vi "show_plot_y_axis.vi"(8 "autoscale":bool=TRUE, 11 "plot_ref_in":refnum<vi>) -> (0 "done":bool, 3 "plot_ref_out":refnum<vi>)   [LabVIEW 2025]
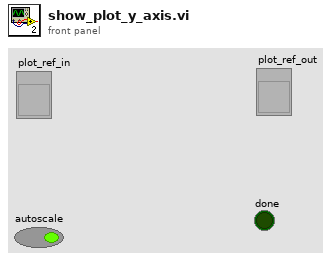
[diagram p1: front panel]
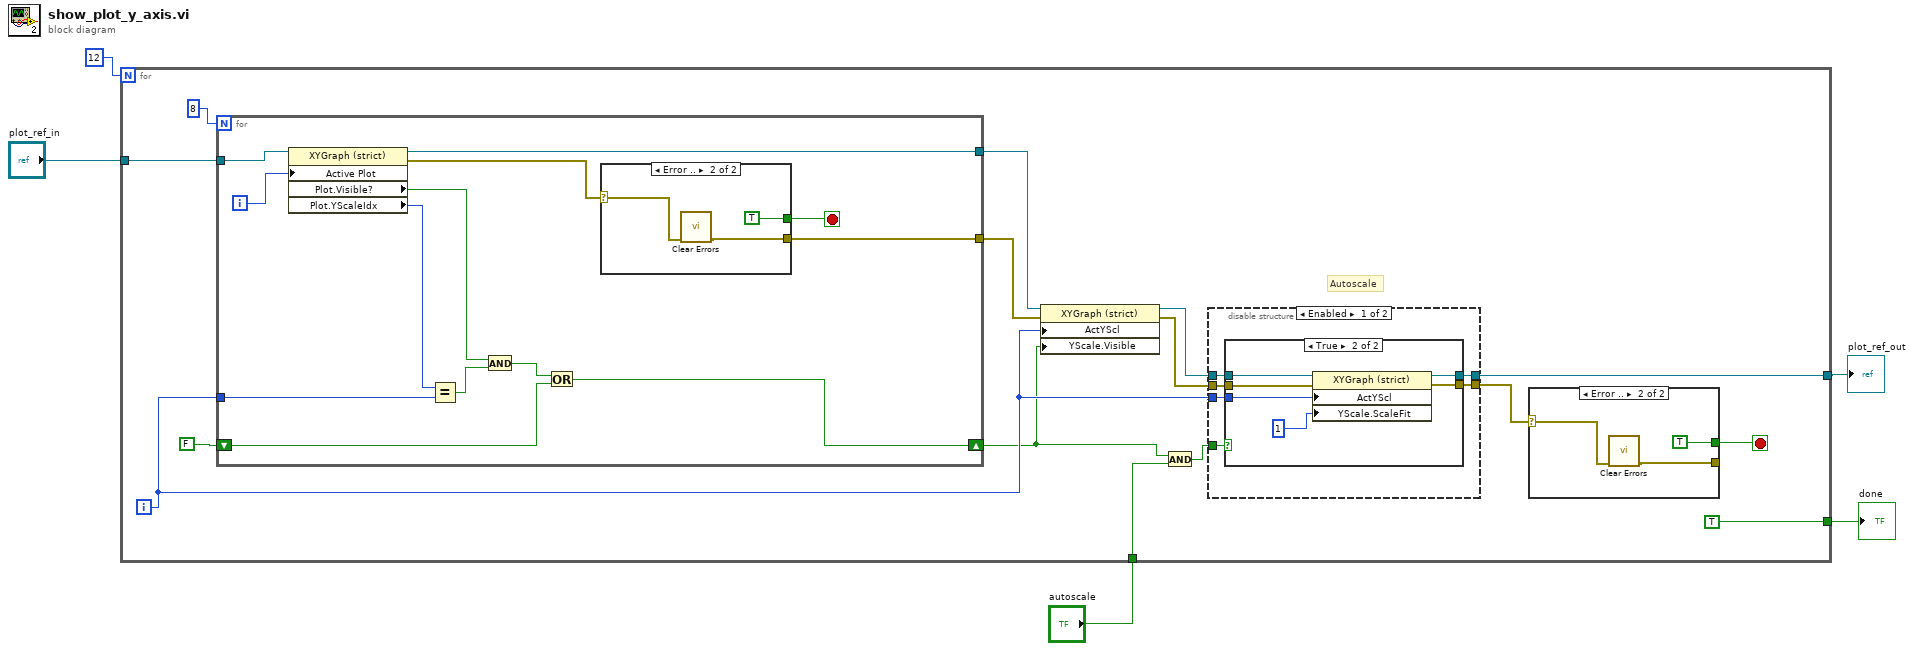
[diagram p0: block diagram]
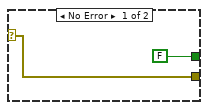
[diagram p4: hidden frame]
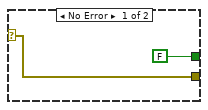
[diagram p5: hidden frame]
diagram:
  n1 = for {
    N: 12 -> [_]
    tunnel: "plot_ref_in" -> [w20]
    tunnel: [TRUE] -> w3
    tunnel: [w9] -> w2
    tunnel: "autoscale" -> [w6]
    i -> [w11]
    stop <- w15 stop-if-true
    # "Autoscale"
    n2 = for {
      N: u32 8 -> [_]
      tunnel: w20 -> [w54]
      tunnel: w11 -> [w46]
      shift-right: [w49] -> w8
      shift-left: FALSE -> [w48]
      tunnel: [w47] -> w18
      tunnel: [w43] -> w17
      i -> [w53]
      stop <- w44 stop-if-true
      n3 = property on="Property Node" class="XYGraph (strict)"(reference=w54, "Active Plot"=w53) -> (reference out=w47:refnum<vi>, error out=w45:errorcluster, "Plot.Visible?"=w51:bool, "Plot.YScaleIdx"=w52:u32)  [unwired: 1 in]
      n4 = Equal?(x=w52, y=w46) -> (x = y?=w50:bool)
      n5 = And(x=w51, y=w50) -> (x .and. y?=w42:bool)
      n6 = Or(x=w42, y=w48) -> (x .or. y?=w49:bool)
      n7 = case shown="Error .." w45 {
        selector: w45 -> [w56 w58]
        tunnel: [FALSE TRUE] -> w44
        tunnel: [w56 w57] -> w43
        frame No Error {
        }
        frame Error {
          n8 = call <vilib>:"Clear Errors.vi"("error in (no error)"=w58) -> ("error out"=w57:errorcluster)  [unwired: 5 in, 1 out]
        }
      }
    }
    n9 = property on="Property Node" class="XYGraph (strict)"(reference=w18, error in=w17, "ActYScl"=w11, "YScale.Visible"=w8) -> (reference out=w13:refnum<vi>, error out=w12:errorcluster)
    n10 = And(x=w8, y=w6) -> (x .and. y?=w7:bool)
    n11 = disable-structure shown="Enabled" {
      disable-tunnel: w7 -> [w26 _]
      disable-tunnel: w13 -> [w25 w35]
      disable-tunnel: w12 -> [w24 w36]
      disable-tunnel: w11 -> [w23 _]
      disable-tunnel: [w22 w36] -> w10
      disable-tunnel: [w21 w35] -> w9
      frame Enabled {
        n12 = case shown="True" w26 {
          tunnel: w25 -> [w27 w34]
          tunnel: w24 -> [w28 w33]
          tunnel: w23 -> [_ w32]
          tunnel: [w28 w30] -> w22
          tunnel: [w27 w29] -> w21
          frame False {
          }
          frame True {
            n13 = property on="Property Node" class="XYGraph (strict)"(reference=w34, error in=w33, "ActYScl"=w32, "YScale.ScaleFit"=u8 1 ("Y Scale.Scale Fit")) -> (reference out=w29:refnum<vi>, error out=w30:errorcluster)
          }
        }
      }
      frame Disabled {
      }
    }
    n14 = case shown="Error .." w10 {
      selector: w10 -> [w38 w40]
      tunnel: [FALSE TRUE] -> w15
      tunnel: [w38 w39] -> _
      frame No Error {
      }
      frame Error {
        n15 = call <vilib>:"Clear Errors.vi"("error in (no error)"=w40) -> ("error out"=w39:errorcluster)  [unwired: 5 in, 1 out]
      }
    }
  }
  "done" <- w3
  "plot_ref_out" <- w2
